vi "findSC.vi"(2 "II channel":i32[][](array[numeric]), 3 "I channel":i32[][](array[numeric])) -> (0 "II channel out":i32[][](array[numeric]), 1 "I channel out":i32[][](array[numeric]))   [LabVIEW 2015]
uses:
  dependecies/globalVarSD.vi
panel:
  out "position":i32
  out "out":dbl[](graph) caption="Data Values"
  out "in":dbl[](graph) caption="Data Values"
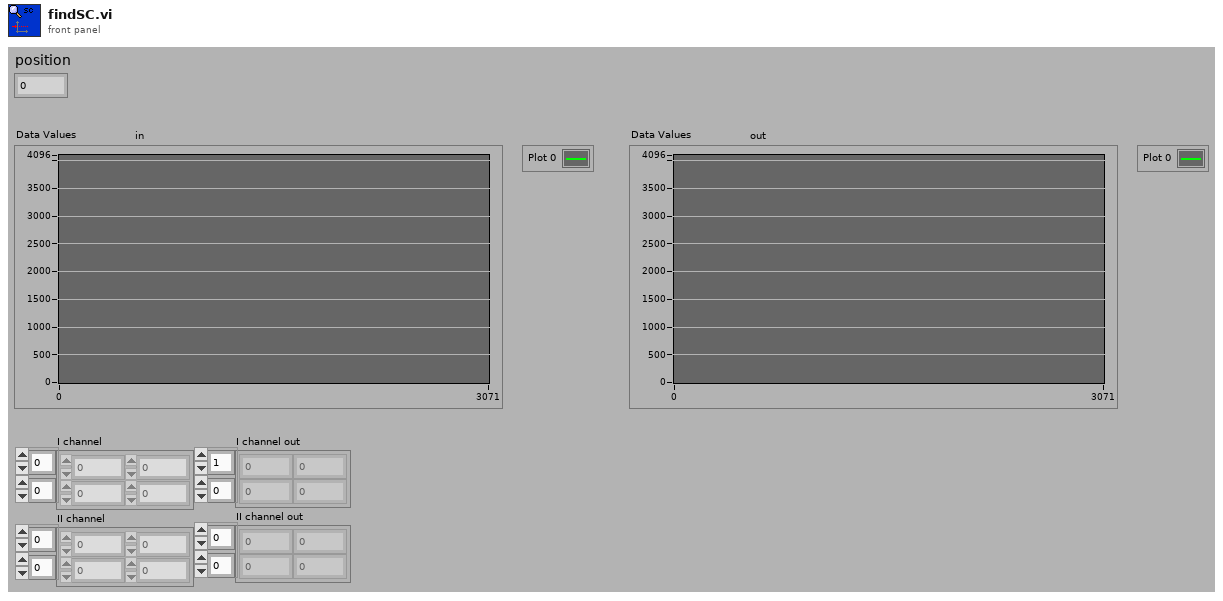
[diagram p1: front panel]
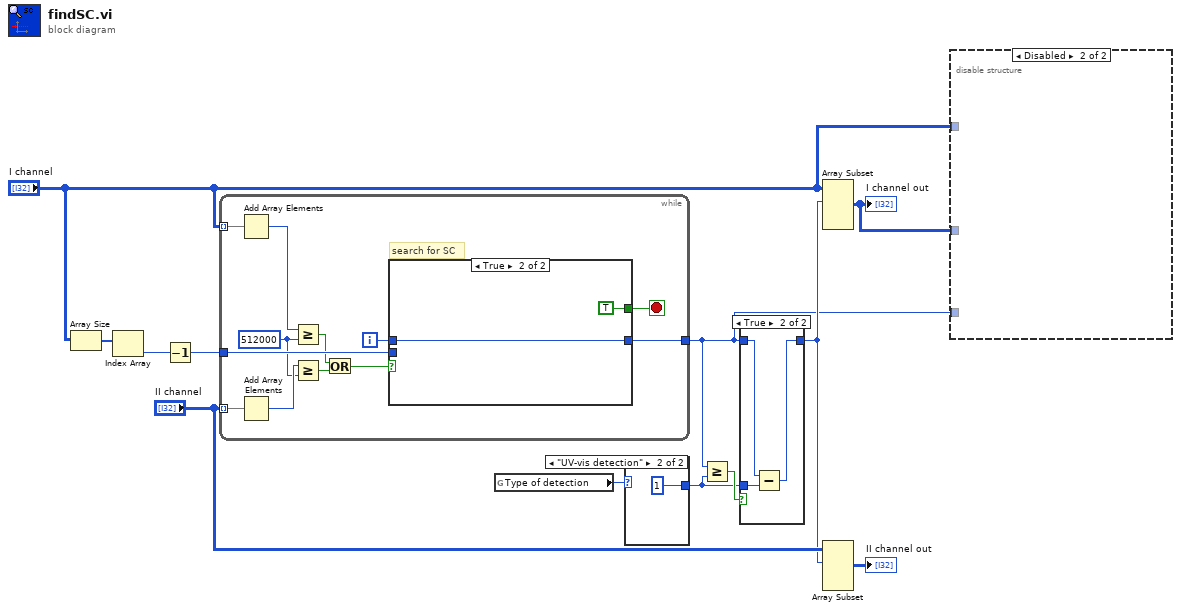
[diagram p0: block diagram]
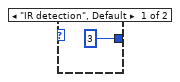
[diagram p2: hidden frame]
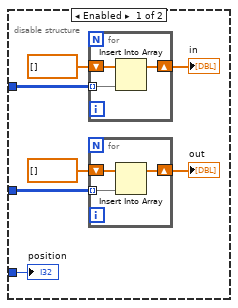
[diagram p4: hidden frame]
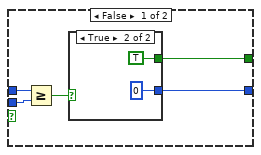
[diagram p5: hidden frame]
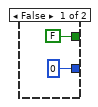
[diagram p6: hidden frame]
diagram:
  n1 = Array Size(array="I channel") -> (size(s)=w7:i32[])
  n2 = Index Array(array=w7) -> (element=w2:i32)  [unwired: 1 in]
  n3 = Decrement(x=w2) -> (x-1=w1:i32)
  n4 = while {
    tunnel: "I channel" -> [w20] mode=indexing
    tunnel: "II channel" -> [w19] mode=indexing
    tunnel: [w23] -> w6
    tunnel: w1 -> [w21]
    i -> [w22]
    stop <- w24 stop-if-true
    w16 = 512000 ("y")
    # "search for SC"
    n5 = Add Array Elements(numeric array=w20) -> (sum=w18:i32)
    n6 = Add Array Elements(numeric array=w19) -> (sum=w17:i32)
    n7 = Greater Or Equal?(x=w18, y=w16) -> (x >= y?=w15:bool)
    n8 = Greater Or Equal?(x=w17, y=w16) -> (x >= y?=w14:bool)
    n9 = Or(x=w15, y=w14) -> (x .or. y?=w13:bool)
    n10 = case shown="True" w13 {
      tunnel: [w26 TRUE] -> w24
      tunnel: [w27 w34] -> w23
      tunnel: w22 -> [w29 w34]
      tunnel: w21 -> [w25 _]
      frame False {
        n11 = Greater Or Equal?(x=w29, y=w25) -> (x >= y?=w28:bool)
        n12 = case shown="True" w28 {
          tunnel: [0 0] -> w27
          tunnel: [FALSE TRUE] -> w26
          frame False {
          }
          frame True {
          }
        }
      }
      frame True {
      }
    }
  }
  n13 = global read "globalVarSD.vi" "Type of detection"() -> (w4:enum32{"IR detection", "UV-vis detection"})
  n14 = case shown="\"UV-vis detection\"" w4 {
    tunnel: [3 ("y") 1 ("y")] -> w3
    frame "IR detection", Default {
    }
    frame "UV-vis detection" {
    }
  }
  n15 = Greater Or Equal?(x=w6, y=w3) -> (x >= y?=w10:bool)
  n16 = case shown="True" w10 {
    tunnel: [w38 w40] -> w9
    tunnel: w6 -> [w38 w41]
    tunnel: w3 -> [_ w39]
    frame False {
    }
    frame True {
      n17 = Subtract(x=w41, y=w39) -> (x-y=w40:i32)
    }
  }
  n18 = Array Subset(array="I channel", index (row)=w9) -> (w5:i32[][])  [unwired: 3 in]
  "I channel out" <- w5
  n19 = Array Subset(array="II channel", index (row)=w9) -> (→"II channel out":i32[][])  [unwired: 3 in]
  n20 = disable-structure shown="Disabled" {
    disable-tunnel: "I channel" -> [w46 _]
    disable-tunnel: w5 -> [w43 _]
    disable-tunnel: w6 -> [w42 _]
    frame Enabled {
      n21 = for {
        tunnel: w46 -> [w52] mode=indexing
        shift-right: [w53] -> w47
        shift-left: dbl[] [] ("tableau") -> [w54]
        n22 = Insert Into Array(array=w54, new element=w52) -> (w53:dbl[])  [unwired: 1 in]
      }
      "in" <- w47
      n23 = for {
        tunnel: w43 -> [w49] mode=indexing
        shift-right: [w50] -> w45
        shift-left: dbl[] [] ("tableau") -> [w51]
        n24 = Insert Into Array(array=w51, new element=w49) -> (w50:dbl[])  [unwired: 1 in]
      }
      "out" <- w45
      "position" <- w42
    }
    frame Disabled {
    }
  }
